vi "Actors Test.vi"() -> ()   [LabVIEW 2020]
uses:
  Test/Actor/Count Behaviour.ctl
  Test/API/Test Actor API.lvclass
  C:/Users/neilp/Desktop/Actors/Actor/API/Actor API.lvclass
  Test/Actor/Test Actor.lvclass
  Base Actor/API/Actor API.lvclass
panel:
  in  "Count Behaviour":T1
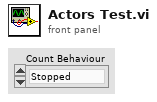
[diagram p1: front panel]
types:
  T1 = typedef "Test Actor.lvclass/Count Behaviour.ctl" = enum16{"Stopped", "Up", "Down"}
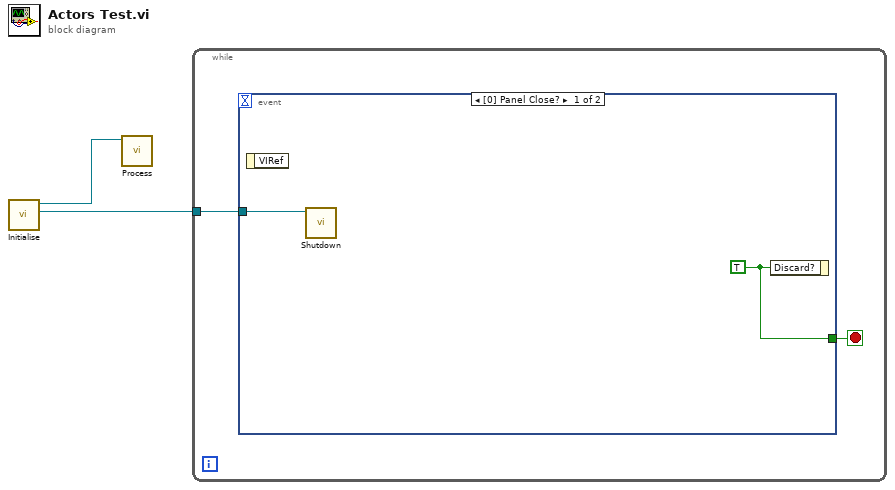
[diagram p0: block diagram]
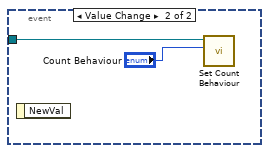
[diagram p2: hidden frame]
diagram:
  n1 = call "Initialise.vi"() -> ("Test Actor API out"=w1:refnum<class "Test Actor API.lvclass">, "Test Actor out"=w2:refnum<class "Test Actor.lvclass">)  [unwired: 9 in, 1 out]
  n2 = call "Process.vi"("Test Actor"=w2) -> ()  [unwired: 11 in]
  n3 = while {
    tunnel: w1 -> [w3]
    stop <- w4 stop-if-true
    n4 = event shown="[0] Panel Close?" {
      selector: _ -> [_ _]
      dyn-events: _ -> [_ _]
      timeout: _ -> [_ _]
      tunnel: [w6 _] -> w4
      tunnel: w3 -> [w5 w8]
      event Panel Close? {
        w6 = TRUE ("Discard?")
        n5 = event-data() -> ()  [unwired: 1 in, 1 out]
        n6 = call "Shutdown.vi"("Actor API in"=w5) -> ()  [unwired: 10 in, 1 out]
        n7 = event-data("Discard?"=w6) -> ()  [unwired: 1 in, 1 out]
      }
      event Value Change {
        n8 = event-data() -> ()  [unwired: 1 in, 1 out]
        n9 = call "Set Count Behaviour.vi"("Count Behaviour"="Count Behaviour", "Test Actor API"=w8) -> ()  [unwired: 9 in, 1 out]
      }
    }
  }
